vi "RegExprTest.vi"() -> ()   [LabVIEW 2013]
panel:
  out "match substring":string
  out "after substring":string
  out "before substring":string
  in  "input string":string
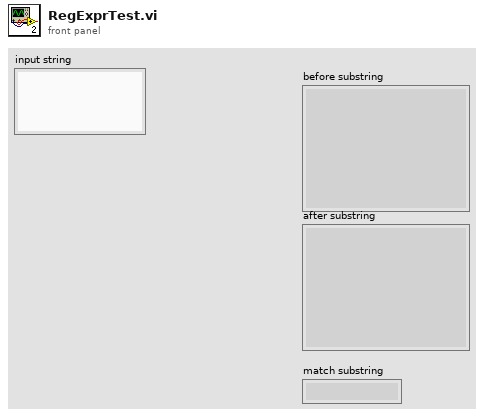
[diagram p1: front panel]
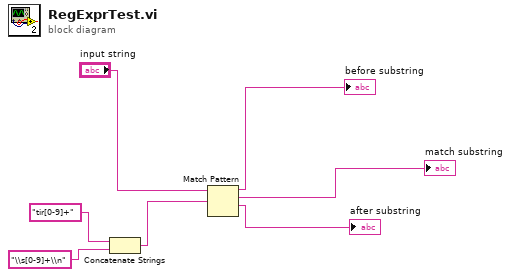
[diagram p0: block diagram]
diagram:
  n1 = Concatenate Strings("tir[0-9]+" ("regular expression"), "\\s[0-9]+\\n" ("regular expression")) -> (w1:string)
  n2 = Match Pattern(string="input string", regular expression=w1) -> (before substring=→"before substring":string, match substring=→"match substring":string, after substring=→"after substring":string)  [unwired: 1 in, 1 out]
